vi "Log to Sinks.vi"(10 "Log Packet":T1, 11 "Asynchronous Application Log in":refnum<class "Application Logger.lvclass">) -> (0 "error out":errorcluster, 3 "Asynchronous Application Log out":refnum<class "Application Logger.lvclass">)   [LabVIEW 2020, in "MVA Framework.lvlib" / "Composed Log.lvlib" / "Application Logger.lvclass"]
uses:
  Application Logger.lvclass
  Types/Log Packet.ctl
  Types/Log Level.ctl
  Application Logger.lvclass/Application Logger.ctl
  Log Sink/Log Sink.lvclass/Log Sink.ctl
  Log Sink/Evaluate Log Packet.vi
  Log Sink/Check Should Log.vi
  Log Sink/Log Sink.lvclass
  ILogFilter/ILogFilter.lvclass
  Composed Log.lvlib
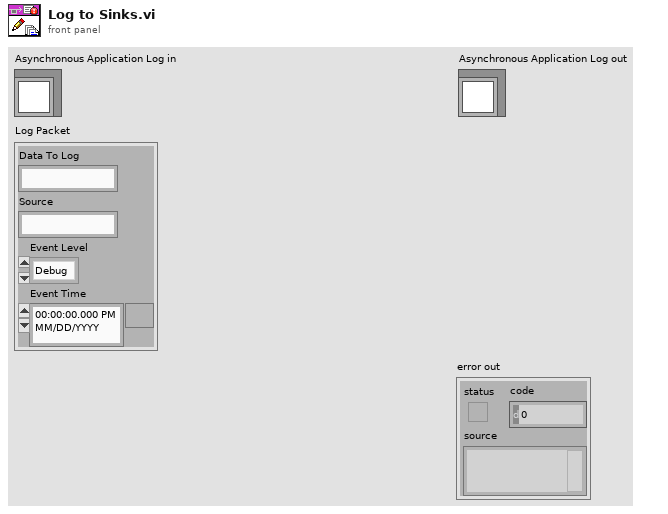
[diagram p1: front panel]
types:
  T1 = typedef "MVA Framework.lvlib/Composed Log.lvlib/Log Packet.ctl" = cluster{"Data To Log":string, "Source":string, "Event Level":T2, "Event Time":timestamp}
  T2 = typedef "MVA Framework.lvlib/Composed Log.lvlib/Log Level.ctl" = enum16{"Debug", "Info", "Warning", "Error", "Critical"}
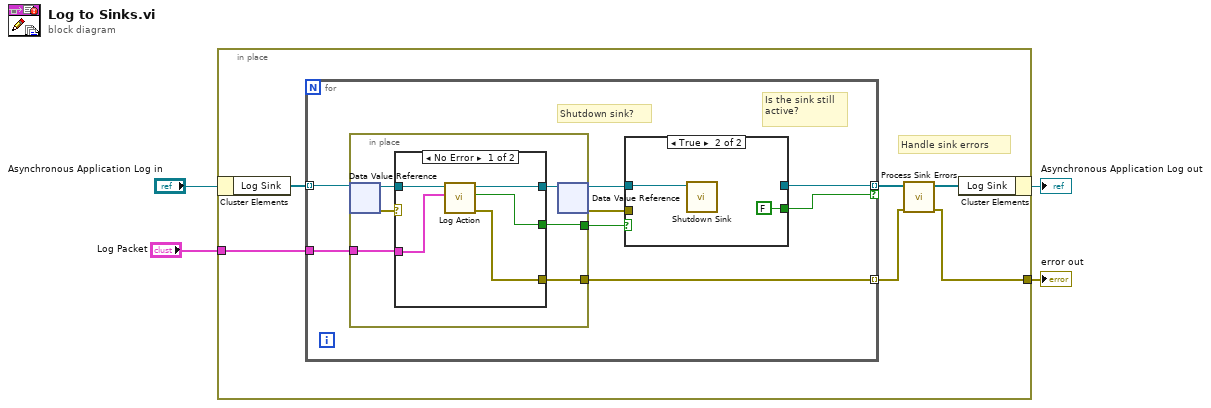
[diagram p0: block diagram]
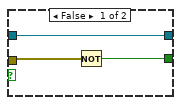
[diagram p2: hidden frame]
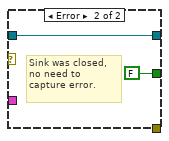
[diagram p3: hidden frame]
diagram:
  n1 = in-place {
    in-place-border: "Log Packet" -> [w9]
    in-place-border: [w5] -> w1
    # "Handle sink errors"
    n2 = in-place-cluster #1("Asynchronous Application Log in") -> ("Log Sink"=w10:refnum<data-value>[])
    n3 = for {
      tunnel: w10 -> [w16] mode=indexing
      tunnel: [w13] -> w8 mode=indexing if=w11
      tunnel: w9 -> [w18]
      tunnel: [w17] -> w6 mode=indexing
      # "Shutdown sink?"
      # "Is the sink still active?"
      n4 = in-place {
        in-place-border: [w26] -> w17
        in-place-border: w18 -> [w25]
        in-place-border: [w24] -> w15
        n5 = in-place-dvr #2(w16) -> (w28:refnum<class "Log Sink.lvclass">, w29:errorcluster)
        n6 = case shown="No Error" w29 {
          tunnel: w28 -> [w34 w36]
          tunnel: [w33 w36] -> w27
          tunnel: [w31 _] -> w26
          tunnel: w25 -> [w32 _]
          tunnel: [w30 FALSE ("Stop Sink?")] -> w24
          frame No Error {
            n7 = call "Log Action.vi"("Log Packet"=w32, "Log Sink in"=w34) -> ("error out"=w31:errorcluster, "Stop Sink?"=w30:bool, "Log Sink out"=w33:refnum<class "Log Sink.lvclass">)  [unwired: 7 in]
          }
          frame Error {
            # "Sink was closed, no need to capture error."
          }
        }
        n8 = in-place-dvr #2(w27) -> (w14:refnum<data-value>, w12:errorcluster)
      }
      n9 = case shown="True" w15 {
        tunnel: w14 -> [w21 w23]
        tunnel: [w21 _] -> w13
        tunnel: w12 -> [w20 _]
        tunnel: [w19 FALSE] -> w11
        frame False {
          n10 = Not(x=w20) -> (.not. x?=w19:bool)
        }
        frame True {
          n11 = call "Shutdown Sink.vi"("Log Sink"=w23) -> ()  [unwired: 10 in, 1 out]
        }
      }
    }
    n12 = call "Process Sink Errors.vi"("error in (no error)"=w6, "Data Sinks In"=w8) -> ("error out"=w5:errorcluster, "Data Sinks Out"=w7:refnum<data-value>[])  [unwired: 8 in]
    n13 = in-place-cluster #1("Log Sink"=w7) -> (→"Asynchronous Application Log out":refnum<class "Application Logger.lvclass">)
  }
  "error out" <- w1
